vi "CRC16 XMODEM.vi"(5 "data":string) -> (2 "crc":string)   [LabVIEW 2021]
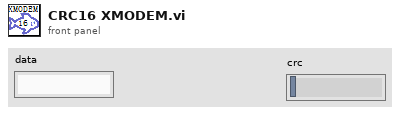
[diagram p1: front panel]
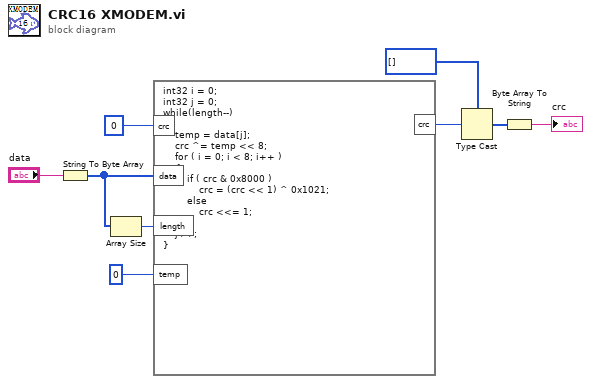
[diagram p0: block diagram]
diagram:
  n1 = String To Byte Array(string="data") -> (unsigned byte array=w8:u8[])
  n2 = Array Size(array=w8) -> (size(s)=w7:i32)
  n3 = formula code="int32 i = 0;\nint32 j = 0;\nwhile(length--)\n{\n    temp = data[j];\n    crc ^= temp << 8; \n    for ( i = 0; i < 8; i++ )\n    {\n        if ( crc & 0x8000 )\n            crc = (crc << 1) ^ 0x1021;\n        else\n            crc <<= 1;\n    }\n    j++;\n}"("data"=w8, "length"=w7, "crc"=u16 0, "temp"=u16 0) -> ("crc"=w4:u16)
  n4 = Type Cast(type=u8[] [] ("unsigned byte array"), x=w4) -> (*(type *) &x=w2:u8[])
  n5 = Byte Array To String(unsigned byte array=w2) -> (string=→"crc":string)
